vi "setPhoneNumbers.vi"(8 "error in (no error)":errorcluster, 10 "phoneNumbers":string[](array[string]), 11 "Shifter in":refnum<class "Shifter.lvclass">) -> (0 "error out":errorcluster, 3 "Shifter out":refnum<class "Shifter.lvclass">)   [LabVIEW 2013, in "Shifter.lvclass"]
uses:
  Shifter.lvclass
  Shifter.lvclass/Shifter.ctl
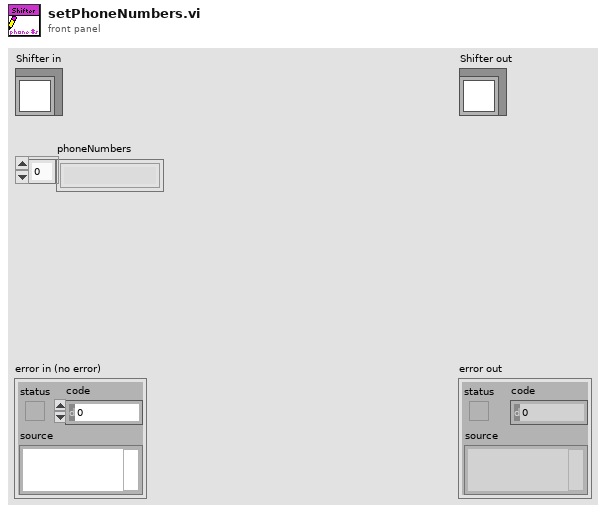
[diagram p1: front panel]
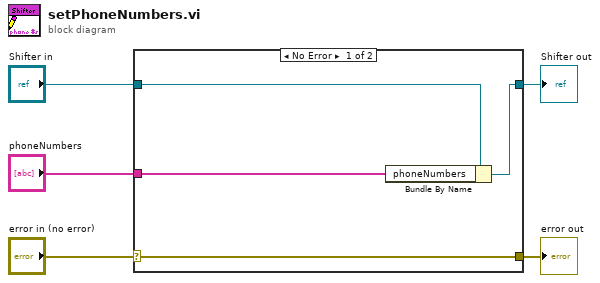
[diagram p0: block diagram]
diagram:
  n1 = case shown="No Error" "error in (no error)" {
    selector: "error in (no error)" -> [w9 w10]
    tunnel: [w9 w10] -> w4
    tunnel: [w7 w11] -> w2
    tunnel: "Shifter in" -> [w8 w11]
    tunnel: "phoneNumbers" -> [w6 _]
    frame No Error {
      n2 = Bundle By Name(cluster=w8, "phoneNumbers"=w6) -> (w7:refnum<class "Shifter.lvclass">)
    }
    frame Error {
    }
  }
  "error out" <- w4
  "Shifter out" <- w2
